vi "KepcoDCPwr Configure Both Voltage Protect Limits.vi"(0 "VISA Session":refnum<visa-resource-name>, 5 "Model In":string, 7 "channel name (\"\")":string="\"\"", 11 "error in (no error)":errorcluster {"code" format="%.0x"}, 12 "limit (0.0)":dbl format="%^.2e", 13 "Neg Limit(0.0)":dbl format="%#_6e") -> (4 "VISA Session Out":refnum<visa-resource-name>, 6 "Model Out":string, 8 "channel name out (\"\")":string="\"\"" caption="channel name Out (\"\")", 15 "error out":errorcluster {"code" format="%.0x"})   [LabVIEW 2010]
doc: "This VI configures the both votlage limits to indepentant values to limit output voltage set points.\n\nThis limit prevents VOLT settings above the limit value. \nNOTE: \nIs identical to Configure Voltage Limits for all products except the BOP 1000W and BOP A."
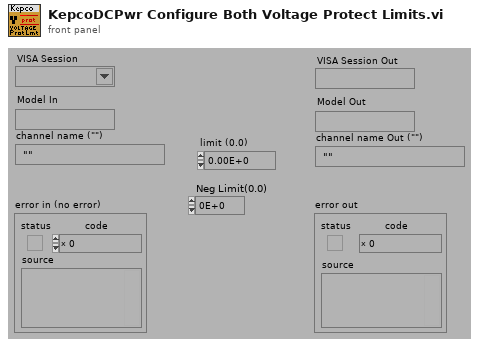
[diagram p1: front panel]
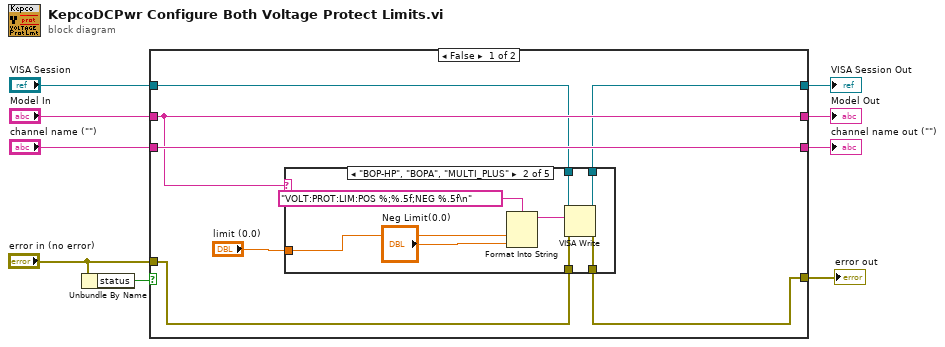
[diagram p0: block diagram]
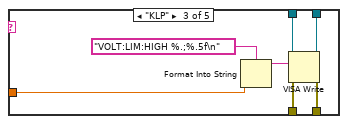
[diagram p3: hidden frame]
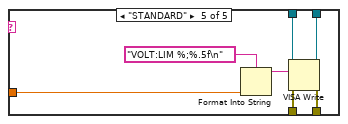
[diagram p5: hidden frame]
diagram:
  n1 = Unbundle By Name("error in (no error)") -> ("status"=w6:bool)
  n2 = case shown="False" w6 {
    tunnel: [w12 w45] -> w9
    tunnel: [w13 w46] -> w7
    tunnel: "VISA Session" -> [w14 w46]
    tunnel: "error in (no error)" -> [w11 w45]
    tunnel: "Model In" -> [w15 w44]
    tunnel: [w15 w44] -> w1
    tunnel: "channel name (\"\")" -> [w16 w43]
    tunnel: [w16 w43] -> w2
    frame False {
      n3 = case shown="\"BOP-HP\", \"BOPA\", \"MULTI_PLUS\"" w15 {
        tunnel: w11 -> [w18 w26 w32 w34 w37]
        tunnel: [w18 w25 w31 w34 w36] -> w12
        tunnel: w14 -> [w17 w24 w33 w35 w39]
        tunnel: [w17 w23 w30 w35 w38] -> w13
        tunnel: "limit (0.0)" -> [_ w21 w27 _ w40]
        frame "", Default {
        }
        frame "BOP-HP", "BOPA", "MULTI_PLUS" {
          n4 = Format Into String(format string="VOLT:PROT:LIM:POS %;%.5f;NEG %.5f\n", w21, "Neg Limit(0.0)") -> (resulting string=w22:string)  [unwired: 2 in, 1 out]
          n5 = VISA Write(VISA resource name=w24, write buffer=w22, error in (no error)=w26) -> (VISA resource name out=w23:refnum<visa-resource-name>, error out=w25:errorcluster)  [unwired: 1 out]
        }
        frame "KLP" {
          n6 = Format Into String(format string="VOLT:LIM:HIGH %.;%.5f\n", w27) -> (resulting string=w28:string)  [unwired: 2 in, 1 out]
          n7 = VISA Write(VISA resource name=w33, write buffer=w28, error in (no error)=w32) -> (VISA resource name out=w30:refnum<visa-resource-name>, error out=w31:errorcluster)  [unwired: 1 out]
        }
        frame "BOP-LP", "MULTI" {
        }
        frame "STANDARD" {
          n8 = Format Into String(format string="VOLT:LIM %;%.5f\n", w40) -> (resulting string=w41:string)  [unwired: 2 in, 1 out]
          n9 = VISA Write(VISA resource name=w39, write buffer=w41, error in (no error)=w37) -> (VISA resource name out=w38:refnum<visa-resource-name>, error out=w36:errorcluster)  [unwired: 1 out]
        }
      }
    }
    frame True {
    }
  }
  "error out" <- w9
  "VISA Session Out" <- w7
  "channel name out (\"\")" <- w2
  "Model Out" <- w1
